vi "error.ExtractErrorMessage.vi"(8 "error in (no error)":errorcluster, 9 "include bold tags? (F)":bool) -> (3 "error message":string)   [LabVIEW 2020]
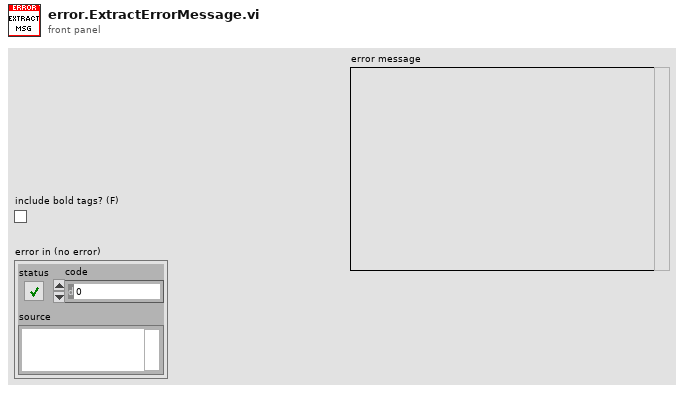
[diagram p1: front panel]
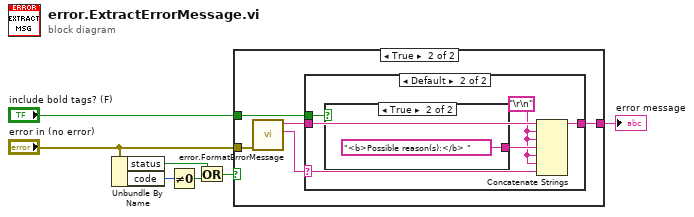
[diagram p0: block diagram]
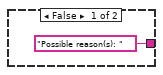
[diagram p4: hidden frame]
diagram:
  n1 = Unbundle By Name("error in (no error)") -> ("status"=w5:bool, "code"=w3:i32)
  n2 = Not Equal To 0?(x=w3) -> (x != 0?=w4:bool)
  n3 = Or(x=w5, y=w4) -> (x .or. y?=w6:bool)
  n4 = case shown="True" w6 {
    tunnel: [_ w12] -> w7
    tunnel: "error in (no error)" -> [_ w11]
    tunnel: "include bold tags? (F)" -> [_ w8]
    frame False {
    }
    frame True {
      n5 = call "error.FormatErrorMessage.vi"("error in (no error)"=w11) -> ("description"=w9:string, "source"=w10:string)  [unwired: 8 in, 1 out]
      n6 = case shown="Default" w9 {
        selector: w9 -> [_ w16]
        tunnel: w10 -> [w13 w19]
        tunnel: [w13 w18] -> w12
        tunnel: w8 -> [_ w14]
        frame "" {
        }
        frame Default {
          w15 = "\r\n" ("End of Line Constant")
          n7 = case shown="True" w14 {
            tunnel: ["Possible reason(s): " ("string") "<b>Possible reason(s):</b> " ("string")] -> w17
            frame False {
            }
            frame True {
            }
          }
          n8 = Concatenate Strings(w19, w15, w15, w17, w15, w15, w16) -> (w18:string)
        }
      }
    }
  }
  "error message" <- w7
